vi "Link Variables.vi"(8 "error in (no error)":errorcluster, 11 "Bus Monitor in":refnum<class "Bus Monitor.lvclass">) -> (0 "error out":errorcluster, 3 "Bus Monitor out":refnum<class "Bus Monitor.lvclass">)   [LabVIEW 2020, in "BCI-1553 API.lvlib" / "Bus Monitor.lvclass"]
doc: "Variable linkage is a bit different for the bus monitor.\n\nBoth Bus A and Bus B will use a special LUT that is exclusive to the bus monitor. This LUT makes the searches for parameters against the command list more efficient. The parameter read table is no longer populated at all. The filters are stored directly in the new tables and have a method for updating and retrieving parameter values.\n\nVariables/parameters get linked to a particular command word. This will be an entry in the command buffer that they will be looking for to identify the valid data fields to use."
uses:
  Bus Monitor.lvclass
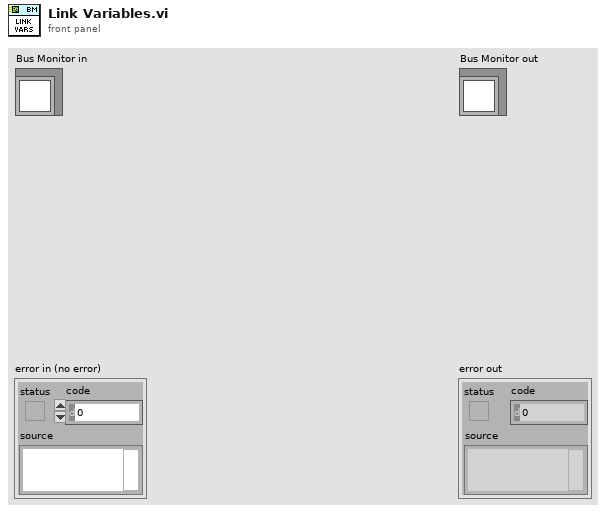
[diagram p1: front panel]
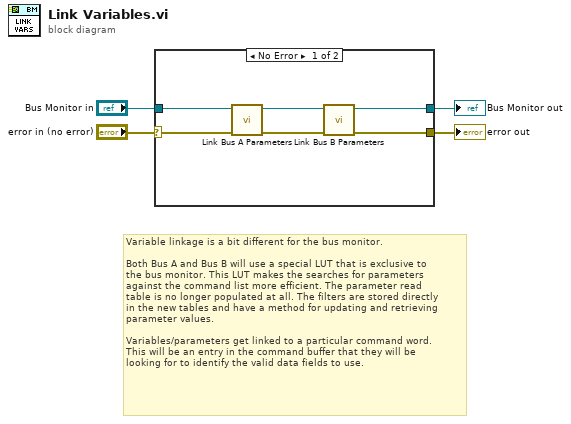
[diagram p0: block diagram]
diagram:
  # "Variable linkage is a bit different for the bus monitor.\n\nBoth Bus A and Bus B will use a special LUT that is exclusive to\nthe bus monitor. This LUT makes the searches for parameters\nagainst the command list more efficient. The parameter read\ntable is no longer populated at all. The filters are stored directly\nin the new tables and have a method for updating and retrieving\nparameter values.\n\nVariables/parameters get linked to a particular command word.\nThis will be an entry in the command buffer that they will be\nlooking for to identify the valid data fields to use."
  n1 = case shown="No Error" "error in (no error)" {
    selector: "error in (no error)" -> [w6 w12]
    tunnel: [w5 w12] -> w3
    tunnel: [w8 w11] -> w1
    tunnel: "Bus Monitor in" -> [w9 w11]
    frame No Error {
      n2 = call "Link Bus A Parameters.vi"("error in (no error)"=w6, "Bus Monitor in"=w9) -> ("error out"=w7:errorcluster, "Bus Monitor out"=w10:refnum<class "Bus Monitor.lvclass">)  [unwired: 8 in]
      n3 = call "Link Bus B Parameters.vi"("error in (no error)"=w7, "Bus Monitor in"=w10) -> ("error out"=w5:errorcluster, "Bus Monitor out"=w8:refnum<class "Bus Monitor.lvclass">)  [unwired: 8 in]
    }
    frame Error {
    }
  }
  "error out" <- w3
  "Bus Monitor out" <- w1
